vi "Set Closed Loop Update Interval.vi"(4 "error in (no error)":errorcluster, 5 "Interval (0 ms)":i32 min=0 max=60000, 6 "Axis (1)":i32=1 min=0 max=3, 7 "VISA resource name":refnum<visa-resource-name>) -> (0 "error out":errorcluster, 3 "VISA resource name out":refnum<visa-resource-name>)   [LabVIEW 2014, in "Newport ESP301.lvlib"]
doc: "This command is used to set the closed loop update interval for an axis. This will be the time duration between position error corrections during closed loop stepper positioning. <B>Note</B> that this command is effective only for steeper motors.\nFurthermore, <B>Note</B> that encoder feedback and closed loop positioning must be enabled for this command to be effective. Refer to feedback configuration (ZB) command for enabling these features in the case of stepper motors.\nIf \"0\" is used as an axis number, this command will set the specified interval to all the axes."
uses:
  Newport ESP301.lvlib
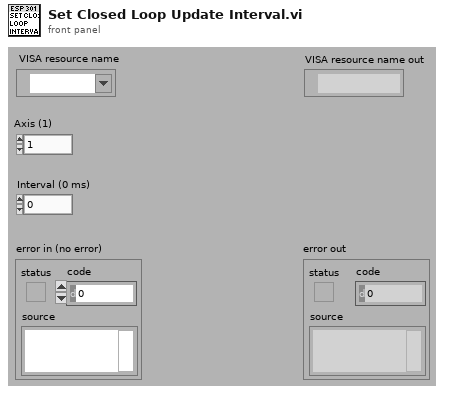
[diagram p1: front panel]
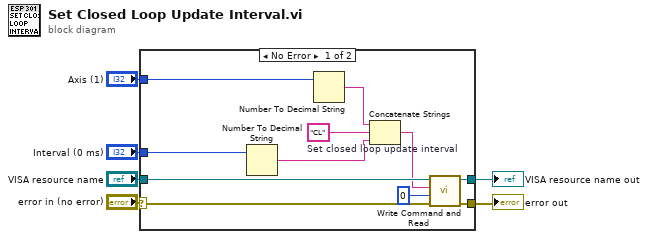
[diagram p0: block diagram]
diagram:
  n1 = case shown="No Error" "error in (no error)" {
    selector: "error in (no error)" -> [w11 w19]
    tunnel: [w9 w19] -> w6
    tunnel: "VISA resource name" -> [w14 w18]
    tunnel: [w10 w18] -> w5
    tunnel: "Axis (1)" -> [w15 _]
    tunnel: "Interval (0 ms)" -> [w7 _]
    frame No Error {
      w17 = "CL"  # Set closed loop update interval
      n2 = Number To Decimal String(number=w7) -> (decimal integer string=w8:string)  [unwired: 1 out]
      n3 = Number To Decimal String(number=w15) -> (decimal integer string=w16:string)  [unwired: 1 out]
      n4 = Concatenate Strings(w16, w17, w8) -> (w13:string)
      n5 = call "Write Command and Read.vi"("error in (no error)"=w11, "Bytes to read (100)"=u32 0, "Command"=w13, "VISA resource name"=w14) -> ("error out"=w9:errorcluster, "VISA resource name out"=w10:refnum<visa-resource-name>)  [unwired: 1 in, 3 out]
    }
    frame Error {
    }
  }
  "error out" <- w6
  "VISA resource name out" <- w5
